vi "replaceVIWithItemFromNewLibrary.vi"(6 "SubVI Path":path, 8 "error in (no error)":errorcluster, 9 "SubVI Refnum":refnum<vi>, 10 "Calling VI Reference":refnum<vi>, 11 "Dependency in":refnum<class "Dependency.lvclass">) -> (0 "error out":errorcluster, 3 "Dependency out":refnum<class "Dependency.lvclass">)   [LabVIEW 2016, in "Dependency.lvclass"]
uses:
  Dependency/Dependency.lvclass
  Dependency/Dependency.lvclass/Dependency.ctl
  Search/Search.lvclass/Search.ctl
  Variables/VIsReplaced.vi
  Variables/VIsReplaceFailed.vi
  Search/Search.lvclass
  Variables/SwitchDependenciesVariables.lvlib
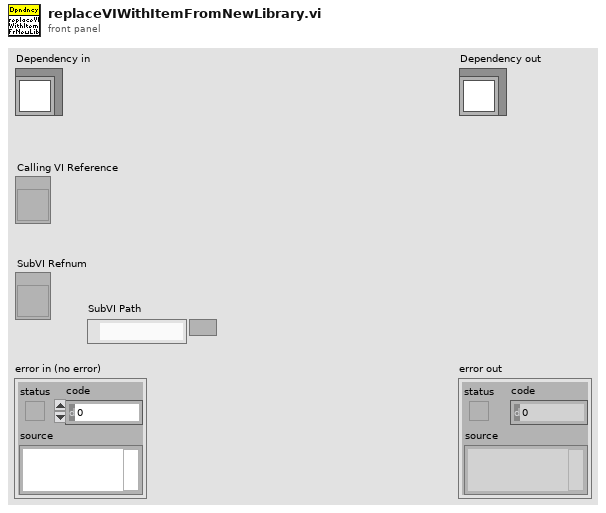
[diagram p1: front panel]
types:
  T1 = typedef "LibraryMemberNameReplacement.ctl" = cluster{"String To Replace in VI names":string, "String To Replace in Control names":string, "New String in VI names":string, "New String in Control names":string}
  T2 = typedef "LibraryDirectories.ctl" = cluster{"OldLibraryDirectory":string, "NewLibraryDirectory":string}
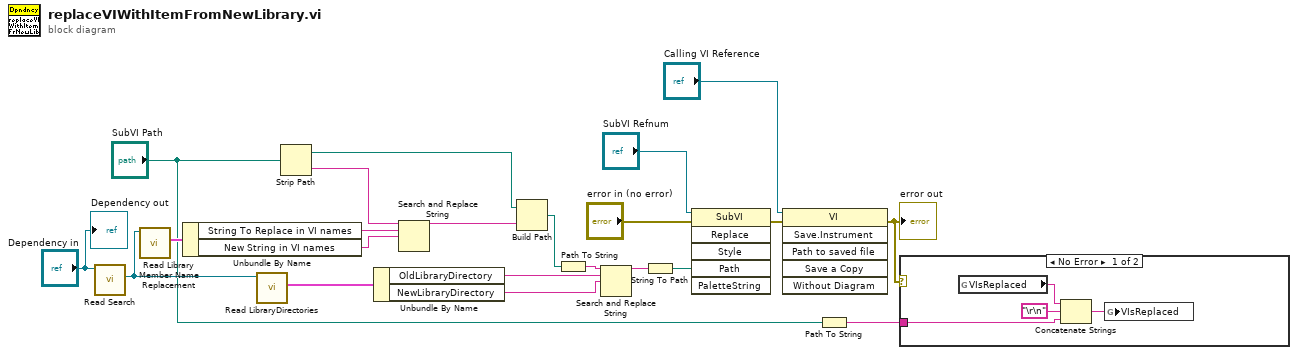
[diagram p0: block diagram]
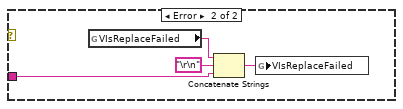
[diagram p2: hidden frame]
diagram:
  n1 = call "Read Search.vi"("Dependency in"="Dependency in") -> ("Search"=w5:refnum<class "Search.lvclass">)  [unwired: 9 in, 1 out]
  n2 = call "Read Library Member Name Replacement.vi"("ProjectItem in"=w5) -> ("Library Member Name Replacement"=w4:T1)  [unwired: 9 in, 1 out]
  n3 = Unbundle By Name(w4) -> ("String To Replace in VI names"=w17:string, "New String in VI names"=w16:string)
  n4 = call "Read LibraryDirectories.vi"("ProjectItem in"=w5) -> ("LibraryDirectories"=w6:T2)  [unwired: 9 in, 1 out]
  n5 = Strip Path(path="SubVI Path") -> (stripped path=w15:path, name=w18:string)
  n6 = Unbundle By Name(w6) -> ("OldLibraryDirectory"=w10:string, "NewLibraryDirectory"=w9:string)
  n7 = Search and Replace String(input string=w18, search string=w17, replace string=w16) -> (result string=w14:string)  [unwired: 5 in, 3 out]
  n8 = Build Path(base path=w15, name or relative path=w14) -> (appended path=w13:path)
  n9 = Path To String(path=w13) -> (string=w12:string)
  n10 = Search and Replace String(input string=w12, search string=w10, replace string=w9) -> (result string=w11:string)  [unwired: 5 in, 3 out]
  n11 = String To Path(string=w11) -> (path=w22:path)
  n12 = invoke class="SubVI" method="Replace"(reference="SubVI Refnum", error in="error in (no error)", "Path"=w22) -> (error out=w20:errorcluster)  [unwired: 3 in, 5 out]
  n13 = invoke class="VI" method="Save.Instrument"(reference="Calling VI Reference", error in=w20) -> (error out=w2:errorcluster)  [unwired: 4 in, 5 out]
  "error out" <- w2
  n14 = Path To String(path="SubVI Path") -> (string=w3:string)
  n15 = case shown="No Error" w2 {
    tunnel: w3 -> [w24 w28]
    frame No Error {
      n16 = global read "VIsReplaced.vi" "VIsReplaced"() -> (w26:string)
      n17 = Concatenate Strings(w26, "\r\n", w24) -> (w23:string)
      n18 = global write "VIsReplaced.vi" "VIsReplaced"(w23) -> ()
    }
    frame Error {
      n19 = global read "VIsReplaceFailed.vi" "VIsReplaceFailed"() -> (w30:string)
      n20 = Concatenate Strings(w30, "\r\n", w28) -> (w27:string)
      n21 = global write "VIsReplaceFailed.vi" "VIsReplaceFailed"(w27) -> ()
    }
  }
  "Dependency out" <- "Dependency in"
